vi "Write List Dqmh Default Events.vi"(8 "error in (no error)":errorcluster, 10 "List Dqmh Default Events":bool, 11 "Lv Proj Document Type:TAF Proj Config in":refnum<class "TAF Proj Config.lvclass">) -> (0 "error out":errorcluster, 3 "Lv Proj Document Type:TAF Proj Config out":refnum<class "TAF Proj Config.lvclass">)   [LabVIEW 2021, in "TAF Proj Document Type.lvlib" / "TAF Proj Config.lvclass"]
uses:
  <vilib>/Wovalab/AntiDoc/Document Type/Add-ons/LabVIEW TAF Project/TAF Proj Config/TAF Proj Config.lvclass
  <vilib>/Wovalab/AntiDoc/Document Type/Add-ons/LabVIEW TAF Project/TAF Proj Config/TAF Proj Config.lvclass/TAF Proj Config.ctl
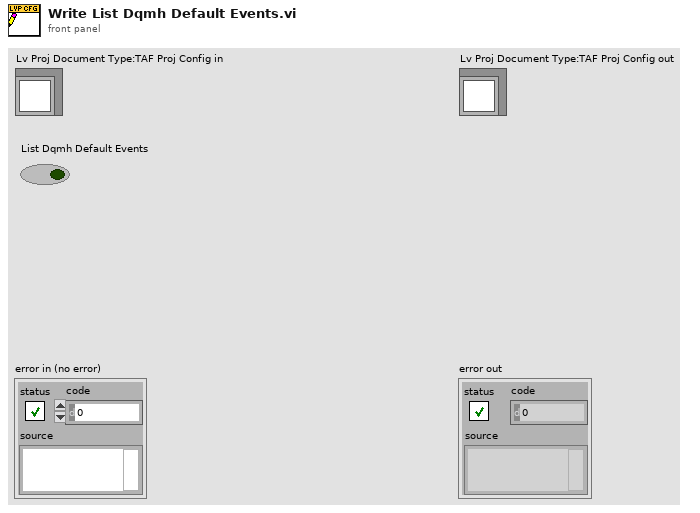
[diagram p1: front panel]
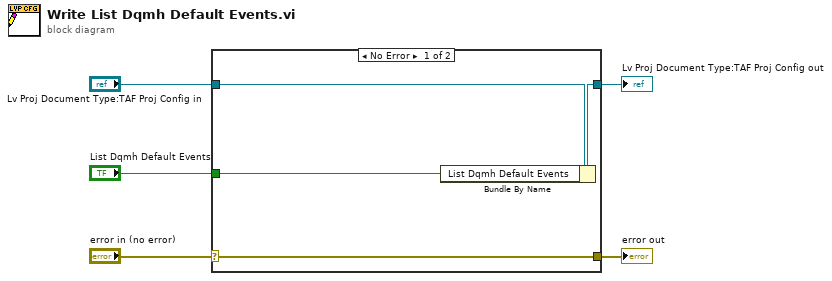
[diagram p0: block diagram]
diagram:
  n1 = case shown="No Error" "error in (no error)" {
    selector: "error in (no error)" -> [w9 w10]
    tunnel: [w9 w10] -> w4
    tunnel: [w7 w11] -> w2
    tunnel: "Lv Proj Document Type:TAF Proj Config in" -> [w8 w11]
    tunnel: "List Dqmh Default Events" -> [w6 _]
    frame No Error {
      n2 = Bundle By Name(cluster=w8, "List Dqmh Default Events"=w6) -> (w7:refnum<class "TAF Proj Config.lvclass">)
    }
    frame Error {
    }
  }
  "error out" <- w4
  "Lv Proj Document Type:TAF Proj Config out" <- w2
